vi "midi_HandleEvent.vi"(7 "event":T1={"status"=0, "channel"=0, "data byte 1"=0, "data byte 2"=0, "tempo"=500000, "track name"="0", "text"=""}, 8 "error in (no error)":errorcluster, 9 "current time (tics)":u32, 10 "note in":u32[][](array[numeric]), 11 "keyboard in":u32[][][](array[numeric])) -> (0 "error out":errorcluster, 2 "note out":u32[][](array[numeric]), 3 "keyboard out":u32[][][](array[numeric]))   [LabVIEW 2013]
doc: "Interpret MIDI events that relate to the production of notes."
panel:
  # "midi_HandleEvent"
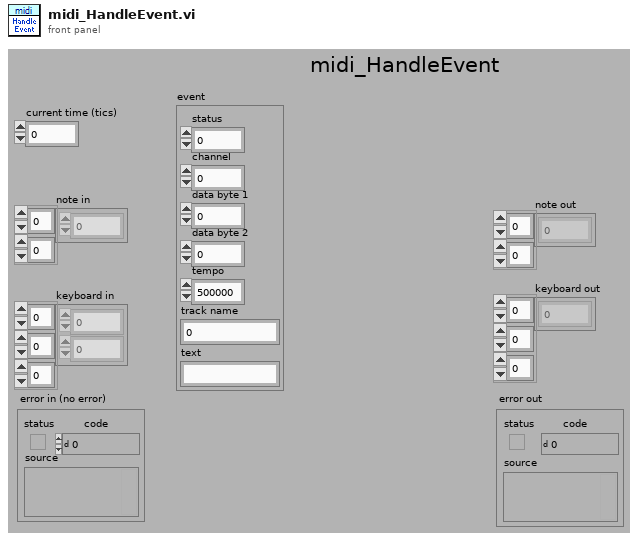
[diagram p1: front panel]
types:
  T1 = cluster{"status":u8, "channel":u8, "data byte 1":u8, "data byte 2":u8, "tempo":u32, "track name":string, "text":string}
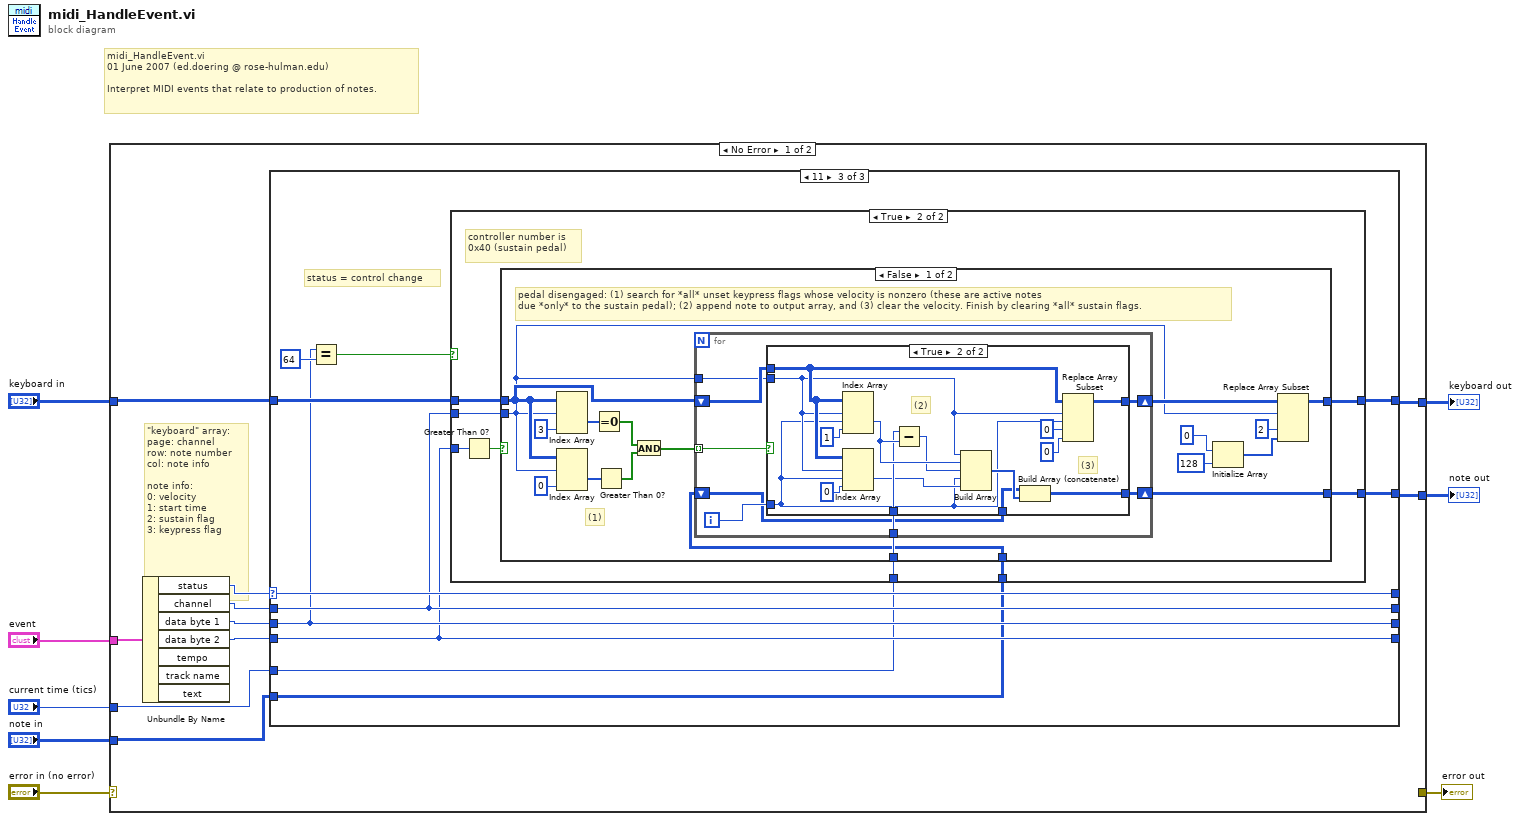
[diagram p0: block diagram]
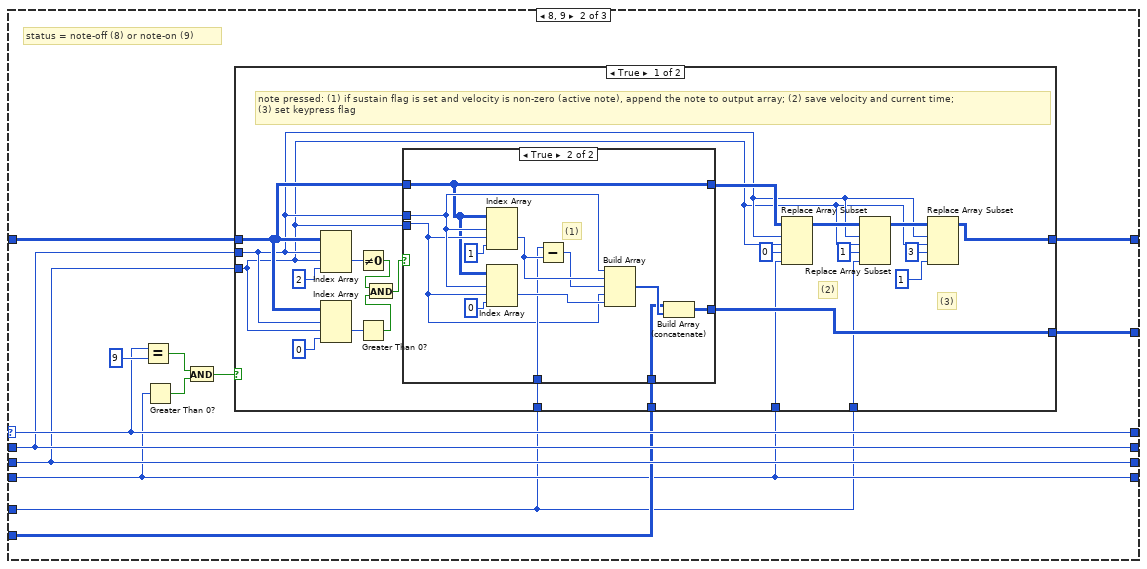
[diagram p3: hidden frame]
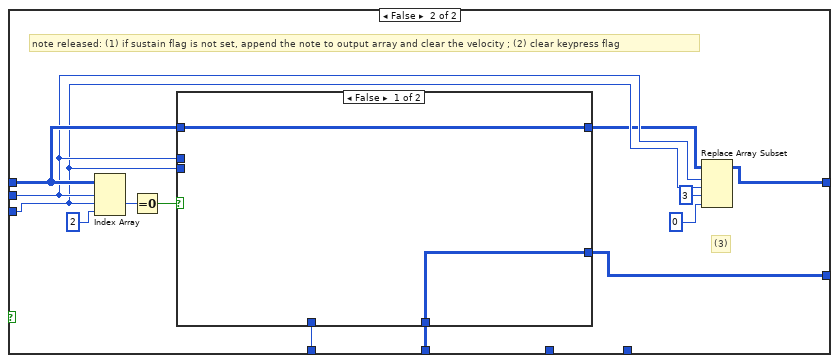
[diagram p5: hidden frame]
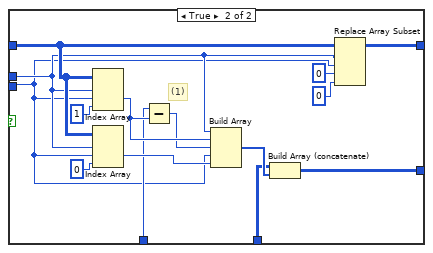
[diagram p6: hidden frame]
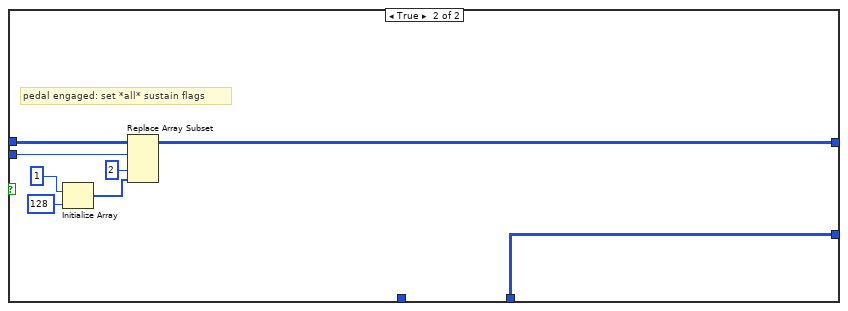
[diagram p9: hidden frame]
diagram:
  # "midi_HandleEvent.vi\n01 June 2007 (ed.doering @ rose-hulman.edu)\n\nInterpret MIDI events that relate to production of notes."
  n1 = case shown="No Error" "error in (no error)" {
    selector: "error in (no error)" -> [_ w177]
    tunnel: [_ w177] -> w7
    tunnel: "keyboard in" -> [w11 _]
    tunnel: "event" -> [w13 _]
    tunnel: "current time (tics)" -> [w12 _]
    tunnel: "note in" -> [w14 _]
    tunnel: [w10 _] -> w2
    tunnel: [w9 _] -> w1
    frame No Error {
      # "\"keyboard\" array:\npage: channel\nrow: note number\ncol: note info\n\nnote info:\n0: velocity\n1: start time\n2: sustain flag\n3: keypress flag"
      n2 = Unbundle By Name(w13) -> ("status"=w15:u8, "channel"=w16:u8, "data byte 1"=w18:u8, "data byte 2"=w17:u8)  [unwired: 3 out]
      n3 = case shown="11" w15 {
        selector: w15 -> [w23 w34 w112]
        tunnel: w18 -> [w21 w30 w110]
        tunnel: w17 -> [w20 w26 w109]
        tunnel: w11 -> [w24 w32 w114]
        tunnel: w16 -> [w22 w31 w111]
        tunnel: [w24 w27 w113] -> w10
        tunnel: [w23 w34 w112] -> _
        tunnel: [w22 w31 w111] -> _
        tunnel: [w21 w30 w110] -> _
        tunnel: [w20 w26 w109] -> _
        tunnel: w12 -> [_ w25 w107]
        tunnel: w14 -> [w19 w29 w106]
        tunnel: [w19 w28 w105] -> w9
        frame 0, Default {
          # "ignore all other events"
        }
        frame 8, 9 {
          # "status = note-off (8) or note-on (9)"
          n4 = Equal?(x=w34, y=u8 9) -> (x = y?=w37:bool)
          n5 = Greater Than 0?(x=w26) -> (x > 0?=w36:bool)
          n6 = And(x=w37, y=w36) -> (x .and. y?=w33:bool)
          n7 = case shown="True" w33 {
            tunnel: w32 -> [w43 w84]
            tunnel: w31 -> [w42 w78]
            tunnel: w30 -> [w41 w77]
            tunnel: w25 -> [w58 w83]
            tunnel: w29 -> [w57 w82]
            tunnel: [w56 w81] -> w28
            tunnel: [w48 w76] -> w27
            tunnel: w26 -> [w47 _]
            tunnel: w25 -> [w46 _]
            frame True {
              # "(3)"
              # "(2)"
              # "note pressed: (1) if sustain flag is set and velocity is non-zero (active note), append the note to output array; (2) save velocity and current time;\n(3) set keypress flag"
              n8 = Index Array(array=w43, index (dim 0)=w42, index (dim 1)=w41, index (dim 2)=2 ("disabled index (col)")) -> (element=w59:u32)
              n9 = Index Array(array=w43, index (dim 0)=w42, index (dim 1)=w41, index (dim 2)=0 ("disabled index (col)")) -> (element=w45:u32)
              n10 = Not Equal To 0?(x=w59) -> (x != 0?=w39:bool)
              n11 = Greater Than 0?(x=w45) -> (x > 0?=w40:bool)
              n12 = And(x=w39, y=w40) -> (x .and. y?=w38:bool)
              n13 = case shown="True" w38 {
                tunnel: w43 -> [w61 w63]
                tunnel: w42 -> [_ w65]
                tunnel: w41 -> [_ w64]
                tunnel: w58 -> [_ w66]
                tunnel: w57 -> [w62 w68]
                tunnel: [w62 w67] -> w56
                tunnel: [w61 w63] -> w49
                frame False {
                }
                frame True {
                  # "(1)"
                  n14 = Index Array(array=w63, index (dim 0)=w65, index (dim 1)=w64, index (dim 2)=1 ("disabled index (col)")) -> (element=w72:u32)
                  n15 = Index Array(array=w63, index (dim 0)=w65, index (dim 1)=w64, index (dim 2)=0 ("disabled index (col)")) -> (element=w70:u32)
                  n16 = Subtract(x=w66, y=w72) -> (x-y=w71:u32)
                  n17 = Build Array(w65, w72, w71, w64, w70) -> (w69:u32[])
                  n18 = Build Array (concatenate)(w68, w69) -> (w67:u32[][])
                }
              }
              n19 = Replace Array Subset(array=w49, new element=w47, index (dim 0)=w42, index (dim 1)=w41, index (dim 2)=0 ("disabled index (col)")) -> (w50:u32[][][])
              n20 = Replace Array Subset(array=w50, new element=w46, index (dim 0)=w42, index (dim 1)=w41, index (dim 2)=1 ("disabled index (col)")) -> (w54:u32[][][])
              n21 = Replace Array Subset(array=w54, new element=u32 1 ("new element/subarray"), index (dim 0)=w42, index (dim 1)=w41, index (dim 2)=3 ("disabled index (col)")) -> (w48:u32[][][])
            }
            frame False {
              # "(3)"
              # "note released: (1) if sustain flag is not set, append the note to output array and clear the velocity ; (2) clear keypress flag"
              n22 = Index Array(array=w84, index (dim 0)=w78, index (dim 1)=w77, index (dim 2)=2 ("disabled index (col)")) -> (element=w86:u32)
              n23 = Equal To 0?(x=w86) -> (x = 0?=w85:bool)
              n24 = case shown="False" w85 {
                tunnel: w84 -> [w88 w93]
                tunnel: w78 -> [_ w92]
                tunnel: w77 -> [_ w91]
                tunnel: w83 -> [_ w96]
                tunnel: w82 -> [w89 w98]
                tunnel: [w89 w97] -> w81
                tunnel: [w88 w90] -> w75
                frame False {
                }
                frame True {
                  # "(1)"
                  n25 = Index Array(array=w93, index (dim 0)=w92, index (dim 1)=w91, index (dim 2)=1 ("disabled index (col)")) -> (element=w102:u32)
                  n26 = Index Array(array=w93, index (dim 0)=w92, index (dim 1)=w91, index (dim 2)=0 ("disabled index (col)")) -> (element=w100:u32)
                  n27 = Subtract(x=w96, y=w102) -> (x-y=w101:u32)
                  n28 = Build Array(w92, w102, w101, w91, w100) -> (w99:u32[])
                  n29 = Build Array (concatenate)(w98, w99) -> (w97:u32[][])
                  n30 = Replace Array Subset(array=w93, new element=u32 0 ("new element/subarray"), index (dim 0)=w92, index (dim 1)=w91, index (dim 2)=0 ("disabled index (col)")) -> (w90:u32[][][])
                }
              }
              n31 = Replace Array Subset(array=w75, new element=u32 0 ("new element/subarray"), index (dim 0)=w78, index (dim 1)=w77, index (dim 2)=3 ("disabled index (col)")) -> (w76:u32[][][])
            }
          }
        }
        frame 11 {
          # "status = control change"
          n32 = Equal?(x=w110, y=u8 64) -> (x = y?=w108:bool)
          n33 = case shown="True" w108 {
            tunnel: w109 -> [_ w125]
            tunnel: w114 -> [w117 w123]
            tunnel: w111 -> [_ w121]
            tunnel: [w117 w122] -> w113
            tunnel: w107 -> [_ w120]
            tunnel: w106 -> [w116 w119]
            tunnel: [w116 w118] -> w105
            frame False {
              # "ignore all other control change\nevents (for now...)"
            }
            frame True {
              # "controller number is\n0x40 (sustain pedal)"
              n34 = Greater Than 0?(x=w125) -> (x > 0?=w124:bool)
              n35 = case shown="False" w124 {
                tunnel: w123 -> [w136 w172]
                tunnel: [w127 w171] -> w122
                tunnel: w121 -> [w126 w170]
                tunnel: w120 -> [w135 _]
                tunnel: w119 -> [w134 w169]
                tunnel: [w133 w169] -> w118
                frame False {
                  # "(1)"
                  # "pedal disengaged: (1) search for *all* unset keypress flags whose velocity is nonzero (these are active notes\ndue *only* to the sustain pedal); (2) append note to output array, and (3) clear the velocity. Finish by clearing *all* sustain flags."
                  n36 = Index Array(array=w136, index (dim 0)=w126, index (dim 2)=3 ("disabled index (col)")) -> (element=w140:u32[])  [unwired: 1 in]
                  n37 = Index Array(array=w136, index (dim 0)=w126, index (dim 2)=0 ("disabled index (col)")) -> (element=w141:u32[])  [unwired: 1 in]
                  n38 = Equal To 0?(x=w140) -> (x = 0?=w139:bool[])
                  n39 = Greater Than 0?(x=w141) -> (x > 0?=w138:bool[])
                  n40 = And(x=w139, y=w138) -> (x .and. y?=w137:bool[])
                  n41 = for {
                    tunnel: w137 -> [w151] mode=indexing
                    tunnel: w126 -> [w149]
                    tunnel: w135 -> [w147]
                    shift-right: [w145] -> w133
                    shift-left: w134 -> [w146]
                    shift-right: [w144] -> w128
                    shift-left: w136 -> [w150]
                    i -> [w148]
                    n42 = case shown="True" w151 {
                      tunnel: w150 -> [w153 w160]
                      tunnel: w149 -> [_ w159]
                      tunnel: w148 -> [_ w158]
                      tunnel: w147 -> [_ w165]
                      tunnel: w146 -> [w152 w154]
                      tunnel: [w152 w161] -> w145
                      tunnel: [w153 w155] -> w144
                      frame False {
                      }
                      frame True {
                        # "(3)"
                        # "(2)"
                        n43 = Index Array(array=w160, index (dim 0)=w159, index (dim 1)=w158, index (dim 2)=1 ("disabled index (col)")) -> (element=w166:u32)
                        n44 = Index Array(array=w160, index (dim 0)=w159, index (dim 1)=w158, index (dim 2)=0 ("disabled index (col)")) -> (element=w163:u32)
                        n45 = Subtract(x=w165, y=w166) -> (x-y=w164:u32)
                        n46 = Build Array(w159, w166, w164, w158, w163) -> (w162:u32[])
                        n47 = Build Array (concatenate)(w154, w162) -> (w161:u32[][])
                        n48 = Replace Array Subset(array=w160, new element=u32 0 ("new element/subarray"), index (dim 0)=w159, index (dim 1)=w158, index (dim 2)=0 ("disabled index (col)")) -> (w155:u32[][][])
                      }
                    }
                  }
                  n49 = Initialize Array(u32 0 ("element"), 128 ("dimension size")) -> (w129:u32[])
                  n50 = Replace Array Subset(array=w128, new element=w129, index (dim 0)=w126, index (dim 2)=2 ("disabled index (col)")) -> (w127:u32[][][])  [unwired: 1 in]
                }
                frame True {
                  # "pedal engaged: set *all* sustain flags"
                  n51 = Initialize Array(u32 1 ("element"), 128 ("dimension size")) -> (w173:u32[])
                  n52 = Replace Array Subset(array=w172, new element=w173, index (dim 0)=w170, index (dim 2)=2 ("disabled index (col)")) -> (w171:u32[][][])  [unwired: 1 in]
                }
              }
            }
          }
        }
      }
    }
    frame Error {
    }
  }
  "error out" <- w7
  "keyboard out" <- w2
  "note out" <- w1
